vi "Initialize by Index.vi"(8 "error in (no error)":errorcluster, 11 "device index":u32) -> (0 "error out":errorcluster, 3 "device handle out":T1)   [LabVIEW 2021, in "RTL-SDR.lvlib"]
uses:
  RTL-SDR.lvlib
  usr/lib64/librtlsdr.so.0
  Controls/Device Handle.ctl
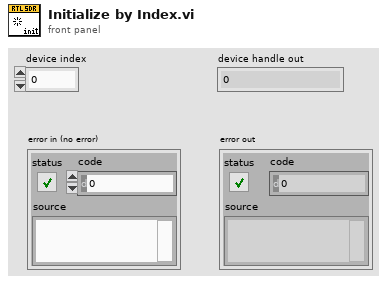
[diagram p1: front panel]
types:
  T1 = typedef "RTL-SDR.lvlib/Device Handle.ctl" = u64
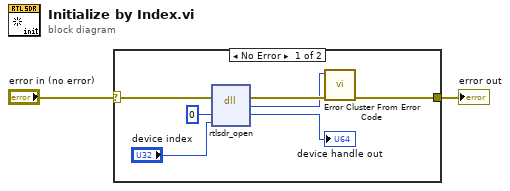
[diagram p0: block diagram]
diagram:
  n1 = case shown="No Error" "error in (no error)" {
    selector: "error in (no error)" -> [w3 w10]
    tunnel: [w6 w10] -> w2
    frame No Error {
      n2 = dll-call lib="usr/lib64/librtlsdr.so.0" fn="rtlsdr_open"(error in=w3, "dev"=u64 0 ("Size"), "index"="device index") -> (error out=w8:errorcluster, "return type"=w7:i32, "dev"=→"device handle out":u64)  [unwired: 3 in, 1 out]
      n3 = call <vilib>:"Error Cluster From Error Code.vi"("error in (no error)"=w8, "error code (0)"=w7) -> ("error out"=w6:errorcluster)  [unwired: 7 in]
    }
    frame Error {
    }
  }
  "error out" <- w2
